vi "Read Nested Queue.vi"(8 "error in (no error)":errorcluster, 10 "Nested Name":string, 11 "Generic Actor in":refnum<class "Generic Actor.lvclass">) -> (0 "error out":errorcluster, 1 "Nested Enqueuer":refnum<class "Message Enqueuer.lvclass">, 2 "not found?":bool, 3 "Generic Actor out":refnum<class "Generic Actor.lvclass">)   [LabVIEW 2020, in "Generic Actor.lvlib" / "Generic Actor.lvclass"]
uses:
  Generic Actor.lvclass
  <vilib>/ActorFramework/Message Enqueuer/Message Enqueuer.lvclass
  Generic Actor.lvclass/Generic Actor.ctl
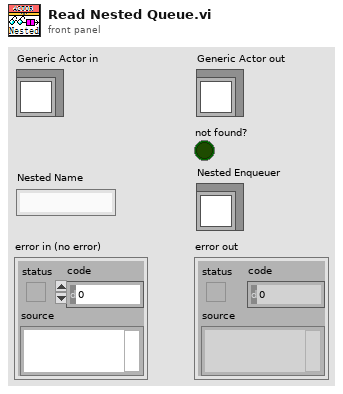
[diagram p1: front panel]
types:
  T1 = map{string, refnum<class "Message Enqueuer.lvclass">}
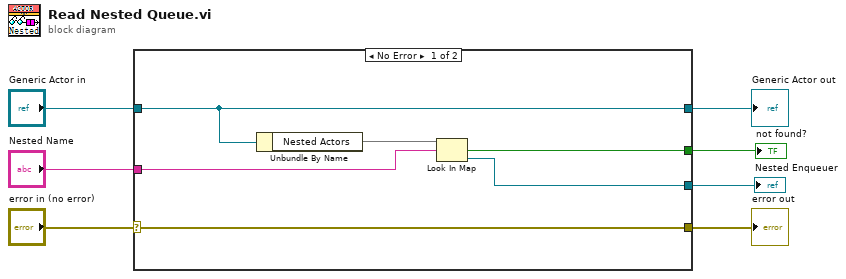
[diagram p0: block diagram]
diagram:
  n1 = case shown="No Error" "error in (no error)" {
    selector: "error in (no error)" -> [w13 w15]
    tunnel: [w13 w15] -> w6
    tunnel: [w12 w14] -> w4
    tunnel: "Generic Actor in" -> [w12 w14]
    tunnel: "Nested Name" -> [w10 _]
    tunnel: [w9 _] -> w2
    tunnel: [w8 _] -> w1
    frame No Error {
      n2 = Unbundle By Name(w12) -> ("Nested Actors"=w11:T1)
      n3 = Look In Map(map=w11, key=w10) -> (key not found?=w8:bool, value=w9:refnum<class "Message Enqueuer.lvclass">)  [unwired: 1 in]
    }
    frame Error {
    }
  }
  "error out" <- w6
  "Generic Actor out" <- w4
  "Nested Enqueuer" <- w2
  "not found?" <- w1
